vi "App.Save.vi"(8 "error in (no error)":errorcluster, 10 "selected path":path, 11 "State Variables":T1={"Aliases.All"=[], "Aliases.Outputs"=[], "UI.Sequence#ofColumns"=0, "SysDef.Path"=path "", "UI.SequenceRef"=refnum, "UI.StepInformationRef"=refnum, "UI.AbortRef"=refnum, "UI.GraphRef"=refnum, "UI.ViewRef"=refnum, "UI.IterationsRef"=refnum, "UI.IterationInformationRef"=refnum, "INI.Settings"={"Build Location"=path "C:/Simple Sequence Editor/SequenceRepo", "LoggingLocation"=path ""}}) -> (0 "error out":errorcluster)   [LabVIEW 2013, in "Simple Sequence Tools - Editor.lvlib"]
uses:
  Simple Sequence Tools - Editor.lvlib
  Types/StateVariables.ctl
  Shared/Types/ChannelProperties.ctl
  Shared/Types/INI.Settings
  Shared/Types/Saved.Sequence.ctl
  Shared/Simple Sequence Tools - Shared.lvlib
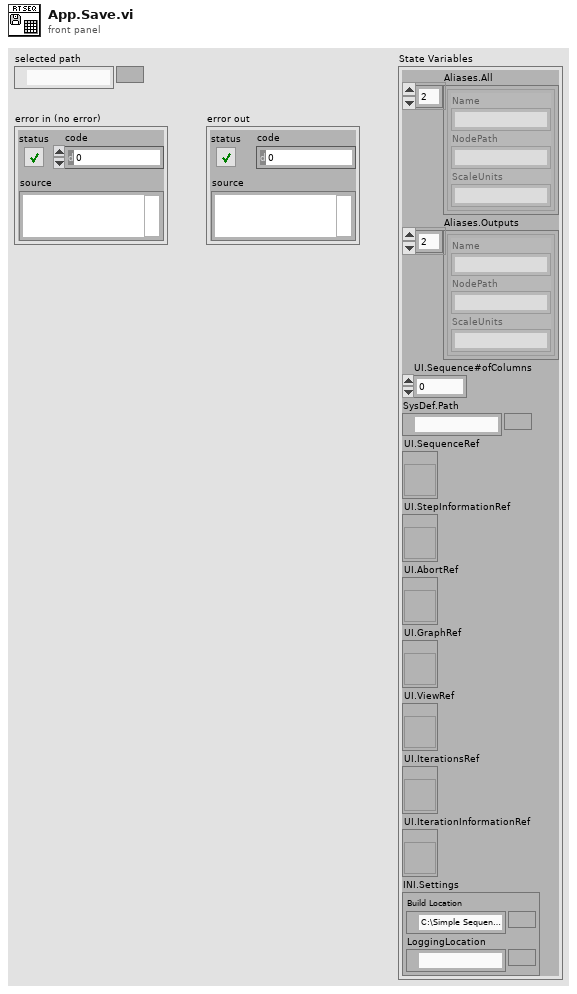
[diagram p1: front panel]
types:
  T1 = typedef "Simple Sequence Tools - Editor.lvlib/StateVariables.ctl" = cluster{"Aliases.All":T2[], "Aliases.Outputs":T2[], "UI.Sequence#ofColumns":i32, "SysDef.Path":path, "UI.SequenceRef":refnum<vi>, "UI.StepInformationRef":refnum<vi>, "UI.AbortRef":refnum<vi>, "UI.GraphRef":refnum<vi>, "UI.ViewRef":refnum<vi>, "UI.IterationsRef":refnum<vi>, "UI.IterationInformationRef":refnum<vi>, "INI.Settings":T3}
  T2 = typedef "Simple Sequence Tools - Shared.lvlib/ChannelProperties.ctl" = cluster{"Name":string, "NodePath":string, "ScaleUnits":string}
  T3 = typedef "Simple Sequence Tools - Shared.lvlib/INI.Settings" = cluster{"Build Location":path, "LoggingLocation":path}
  T4 = typedef "Simple Sequence Tools - Shared.lvlib/Saved.Sequence.ctl" = cluster{"Output Channels":T2[], "Item Names":string[][], "Step":string, "Abort":string, "Iterations":u32, "Iteration":string}
  T5 = enum16{"open", "replace", "create", "open or create", "replace or create", "replace or create with confirmation"}
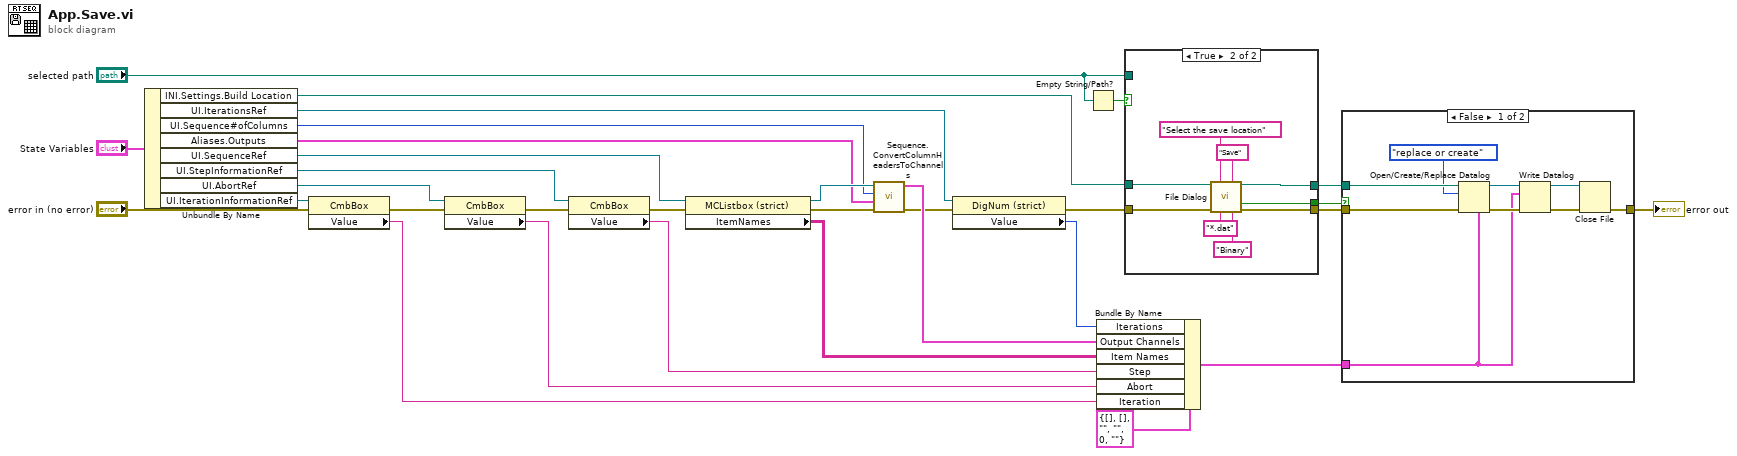
[diagram p0: block diagram]
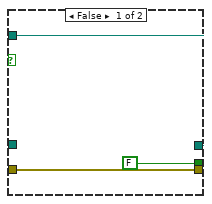
[diagram p2: hidden frame]
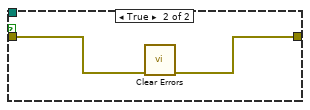
[diagram p3: hidden frame]
diagram:
  n1 = Unbundle By Name("State Variables") -> ("INI.Settings.Build Location"=w1:path, "UI.IterationsRef"=w16:refnum<vi>, "UI.Sequence#ofColumns"=w8:i32, "Aliases.Outputs"=w7:T2[], "UI.SequenceRef"=w17:refnum<vi>, "UI.StepInformationRef"=w23:refnum<vi>, "UI.AbortRef"=w24:refnum<vi>, "UI.IterationInformationRef"=w15:refnum<vi>)
  n2 = property class="CmbBox"(reference=w15, error in="error in (no error)") -> (error out=w13:errorcluster, "Value"=w5:string)  [unwired: 1 out]
  n3 = property class="CmbBox"(reference=w24, error in=w13) -> (error out=w25:errorcluster, "Value"=w30:string)  [unwired: 1 out]
  n4 = property class="CmbBox"(reference=w23, error in=w25) -> (error out=w26:errorcluster, "Value"=w29:string)  [unwired: 1 out]
  n5 = property class="MCListbox (strict)"(reference=w17, error in=w26) -> (reference out=w9:refnum<vi>, error out=w12:errorcluster, "ItemNames"=w4:string[][])
  n6 = call "Sequence.ConvertColumnHeadersToChannels.vi"("error in (no error)"=w12, "Aliases.Outputs"=w7, "UI.Sequence#ofColumns"=w8, "UI.SequenceRef"=w9) -> ("error out"=w11:errorcluster, "Output Channels"=w28:T2[])  [unwired: 5 in, 1 out]
  n7 = property class="DigNum (strict)"(reference=w16, error in=w11) -> (error out=w10:errorcluster, "Value"=w6:u32)  [unwired: 1 out]
  n8 = Empty String/Path?(string/path="selected path") -> (empty?=w3:bool)
  n9 = Bundle By Name(cluster=T4 {"Output Channels"=[], "Item Names"=[], "Step"="", "Abort"="", "Iterations"=0, "Iteration"=""}, "Iterations"=w6, "Output Channels"=w28, "Item Names"=w4, "Step"=w29, "Abort"=w30, "Iteration"=w5) -> (w31:T4)
  n10 = case shown="True" w3 {
    tunnel: [FALSE ("cancelled") w42] -> w21
    tunnel: [w32 w41] -> w20
    tunnel: [w34 w37] -> w19
    tunnel: w10 -> [w34 w35]
    tunnel: "selected path" -> [w32 _]
    tunnel: w1 -> [_ w36]
    frame False {
    }
    frame True {
      n11 = call "File Dialog"("start path"=w36, "prompt"="Select the save location", "button label"="Save", "error in"=w35, "pattern (all files)"="*.dat", "pattern label"="Binary") -> ("selected path"=w41:path, "cancelled"=w42:bool, "error out"=w37:errorcluster)  [unwired: 6 in, 1 out]
    }
  }
  n12 = case shown="False" w21 {
    tunnel: [w52 w53] -> w18
    tunnel: w19 -> [w49 w54]
    tunnel: w20 -> [w51 _]
    tunnel: w31 -> [w45 _]
    frame False {
      n13 = Open/Create/Replace Datalog(5:w45, 8:w49, 10:T5."replace or create" ("operation (0:open)"), 11:w51) -> (0:w48:errorcluster, 3:w46:refnum<k1>)  [unwired: 2 in, 1 out]
      n14 = Write Datalog(4:w48, 6:w45, 7:w46) -> (0:w47:errorcluster, 3:w44:refnum<k1>)
      n15 = Close File(refnum=w44, error in=w47) -> (error out=w52:errorcluster)  [unwired: 1 out]
    }
    frame True {
      n16 = call <vilib>:"Clear Errors.vi"("error in (no error)"=w54) -> ("error out"=w53:errorcluster)  [unwired: 6 in]
    }
  }
  "error out" <- w18
